vi "时间合并-8.6.vi"(0 "年":u8, 1 "月":u8, 2 "日":u8, 3 "时":u8, 4 "分":u8, 5 "秒":u8) -> (13 "秒":string, 14 "年":string, 15 "月":string, 16 "日":string, 17 "时":string, 18 "分":string, 19 "时间":string)   [LabVIEW 2013]
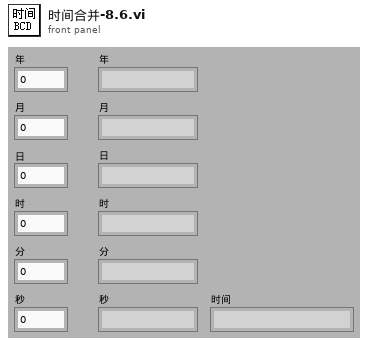
[diagram p1: front panel]
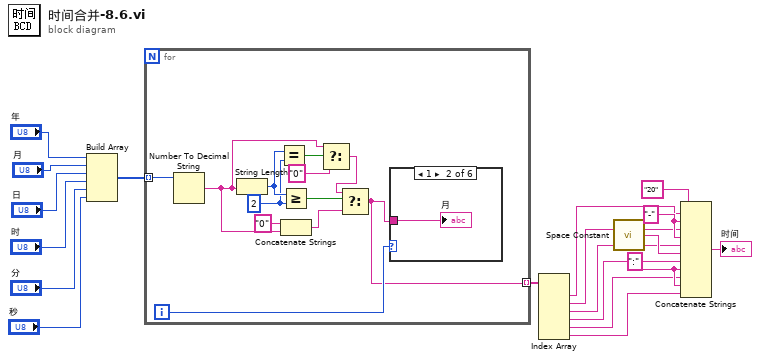
[diagram p0: block diagram]
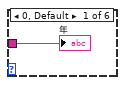
[diagram p2: hidden frame]
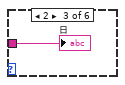
[diagram p3: hidden frame]
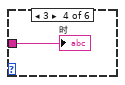
[diagram p4: hidden frame]
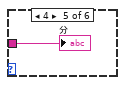
[diagram p5: hidden frame]
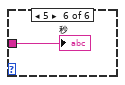
[diagram p6: hidden frame]
diagram:
  w9 = ":" ("字符串")
  w10 = "-" ("字符串")
  n1 = Build Array("年", "月", "日", "时", "分", "秒") -> (w13:u8[])
  n2 = for {
    tunnel: w13 -> [w30] mode=indexing
    tunnel: [w26] -> w7 mode=indexing
    i -> [w31]
    w24 = 2 ("y")
    n3 = Number To Decimal String(number=w30) -> (decimal integer string=w22:string)  [unwired: 1 out]
    n4 = String Length(string=w22) -> (length=w25:i32)
    n5 = Equal?(x=w25, y=w24) -> (x = y?=w23:bool)
    n6 = Greater Or Equal?(x=w25, y=w24) -> (x >= y?=w29:bool)
    n7 = Concatenate Strings("0" ("字符串"), w22) -> (w27:string)
    n8 = Select(t=w22, s=w23, f="0") -> (s? t:f=w21:string)
    n9 = Select(t=w21, s=w29, f=w27) -> (s? t:f=w26:string)
    n10 = case shown="1" w31 {
      tunnel: w26 -> [w32 w33 w34 w35 w36 w37]
      frame 0, Default {
        "年" <- w32
      }
      frame 1 {
        "月" <- w33
      }
      frame 2 {
        "日" <- w34
      }
      frame 3 {
        "时" <- w35
      }
      frame 4 {
        "分" <- w36
      }
      frame 5 {
        "秒" <- w37
      }
    }
  }
  n11 = Index Array(array=w7) -> (element #1=w6:string, element #2=w5:string, element #3=w4:string, element #4=w3:string, element #5=w2:string, element #6=w1:string)  [unwired: 6 in]
  n12 = call <vilib>:"Space Constant.vi"() -> ("String"=w12:string)
  n13 = Concatenate Strings("20" ("字符串"), w6, w10, w5, w10, w4, w12, w3, w9, w2, w9, w1) -> (→"时间":string)
